vi "rrr.vi"() -> ()   [LabVIEW 2016]
panel:
  in  "Knob":dbl(knob) scale=0.0..10.0
  in  "Stop Button":bool
  # "host"
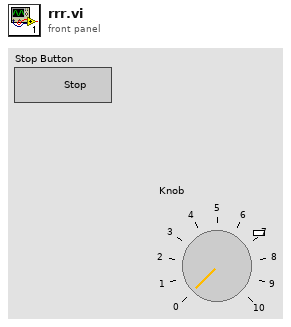
[diagram p1: front panel]
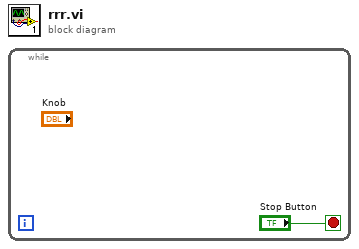
[diagram p0: block diagram]
diagram:
  n1 = while {
    stop <- "Stop Button" stop-if-true
  }
